vi "init.vi"(8 "error in (no error)":errorcluster, 11 "Coffee Actor in":refnum<class "Coffee Actor.lvclass">) -> (0 "error out":errorcluster, 3 "Coffee Actor out":refnum<class "Coffee Actor.lvclass">)   [LabVIEW 2019, in "Coffee Actor.lvlib" / "Coffee Actor.lvclass"]
uses:
  Coffee Actor.lvclass
  Coffee Actor.lvclass/Coffee Actor.ctl
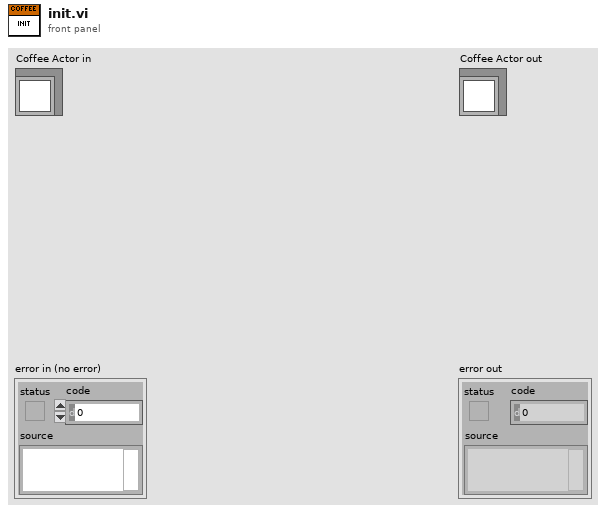
[diagram p1: front panel]
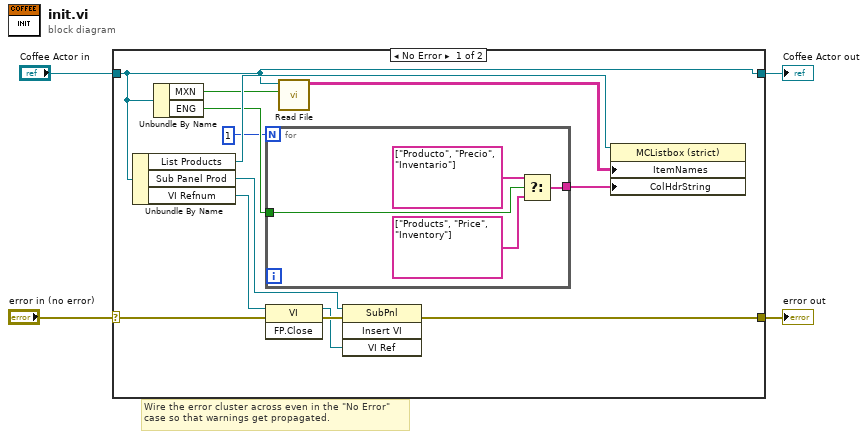
[diagram p0: block diagram]
diagram:
  # "Wire the error cluster across even in the \"No Error\"\ncase so that warnings get propagated."
  n1 = case shown="No Error" "error in (no error)" {
    selector: "error in (no error)" -> [w13 w23]
    tunnel: [w12 w23] -> w3
    tunnel: [w8 w22] -> w1
    tunnel: "Coffee Actor in" -> [w8 w22]
    frame No Error {
      n2 = Unbundle By Name(w8) -> ("List Products"=w11:refnum<vi>, "Sub Panel Prod"=w17:refnum<vi>, "VI Refnum"=w15:refnum<vi>)
      n3 = Unbundle By Name(w8) -> ("MXN"=w7:bool, "ENG"=w6:bool)
      n4 = for {
        N: 1 -> [_]
        tunnel: [w18] -> w10
        tunnel: w6 -> [w21]
        n5 = Select(t=string[] ["Producto", "Precio", "Inventario"] ("Column Header Strings[]"), s=w21, f=string[] ["Products", "Price", "Inventory"] ("Column Header Strings[]")) -> (s? t:f=w18:string[])
      }
      n6 = invoke class="VI" method="FP.Close"(reference=w15, error in=w13) -> (reference out=w14:refnum<vi>, error out=w16:errorcluster)  [unwired: 1 in, 1 out]
      n7 = call "Read File.vi"("MXN"=w7, "Coffee Actor in"=w8) -> ("Array"=w9:string[][])  [unwired: 9 in]
      n8 = invoke class="SubPnl" method="Insert VI"(reference=w17, error in=w16, "VI Ref"=w14) -> (error out=w12:errorcluster)  [unwired: 1 in, 3 out]
      n9 = property class="MCListbox (strict)"(reference=w11, "ItemNames"=w9, "ColHdrString"=w10) -> ()  [unwired: 1 in, 2 out]
    }
    frame Error {
    }
  }
  "error out" <- w3
  "Coffee Actor out" <- w1
